vi "OnDataChange.vi"(0 "Laser_Oxxius in":refnum<class "Laser_Oxxius.lvclass">, 1 "DataExchange":T1, 3 "error in (no error)":errorcluster) -> (7 "Laser_Oxxius out":refnum<class "Laser_Oxxius.lvclass">, 10 "error out":errorcluster)   [LabVIEW 2020]
uses:
  Hardware Abstraction Layer/Component/Device/Device/DataExchange.ctl
  Interface/DataListener/DataListener.lvclass
  Laser_Oxxius.lvclass
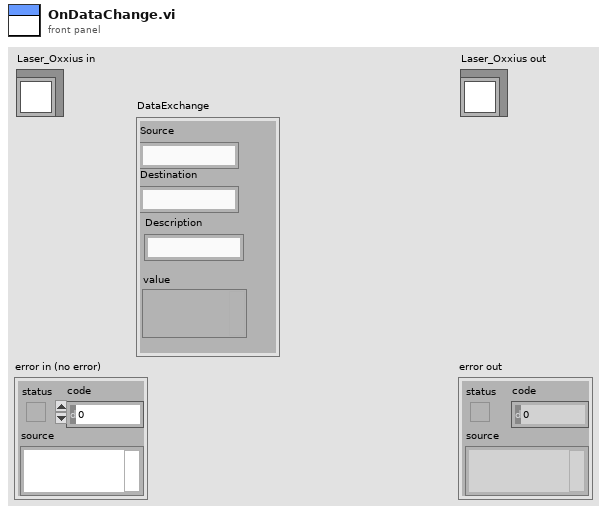
[diagram p1: front panel]
types:
  T1 = typedef "DataListener.lvclass/DataExchange.ctl" = cluster{"Source":string, "Destination":string, "Description":string, "value":variant}
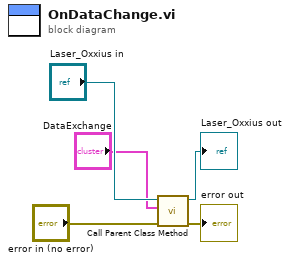
[diagram p0: block diagram]
diagram:
  n1 = call-parent "Call Parent Class Method"("Device in"="Laser_Oxxius in", "DataExchange"="DataExchange", "error in (no error)"="error in (no error)") -> ("Device out"=→"Laser_Oxxius out":refnum<class "Laser_Oxxius.lvclass">, "error out"=→"error out":errorcluster)  [unwired: 6 in]
